vi "Create_AO_Z_WF.vi"(8 "error in":errorcluster) -> (0 "error out":errorcluster)   [LabVIEW 2025]
uses:
  <vilib>/Waveform/WDTOps.llb/WDT Append Waveforms DBL.vi
panel:
  out "Illumination analog waveforms":waveform(dbl)(graph) caption="Output Waveform"
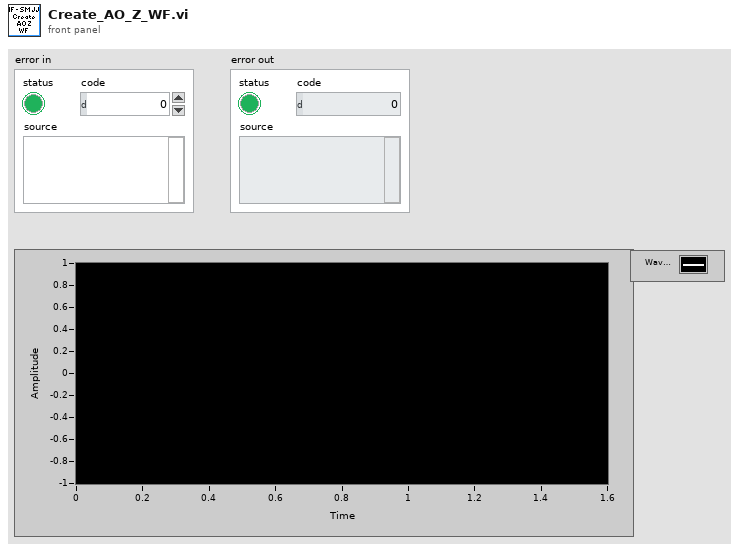
[diagram p1: front panel]
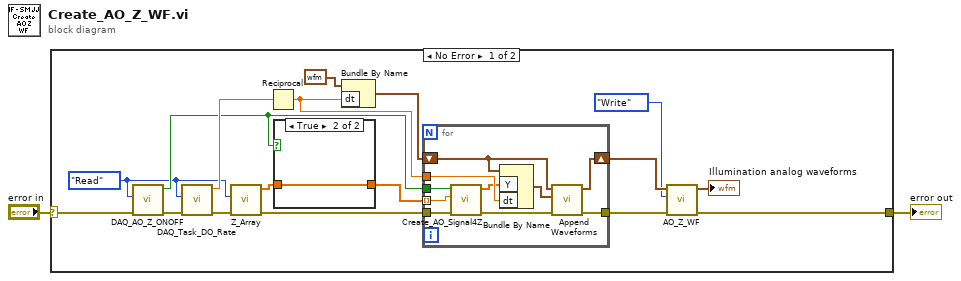
[diagram p0: block diagram]
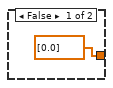
[diagram p2: hidden frame]
diagram:
  n1 = case shown="No Error" "error in" {
    selector: "error in" -> [w19 w32]
    tunnel: [w18 w32] -> w1
    frame No Error {
      w5 = enum16{"Init", "Write", "Read"}."Read" ("Action")
      n2 = call "DAQ_AO_Z_ONOFF.vi"("error in"=w19, "Action"=w5) -> ("error out"=w17:errorcluster, "ON / OFF"=w6:bool)  [unwired: 8 in]
      n3 = call "DAQ_Task_DO_Rate.vi"("error in"=w17, "Action"=w5) -> ("error out"=w9:errorcluster, "DO_Rate"=w16:dbl)  [unwired: 8 in]
      n4 = call "Z_Array.vi"("error in"=w9, "Action"=w5) -> ("error out"=w3:errorcluster, "Z_Array"=w7:dbl[])  [unwired: 8 in]
      n5 = Reciprocal(x=w16) -> (1/x=w13:dbl)
      n6 = case shown="True" w6 {
        tunnel: w7 -> [_ w21]
        tunnel: [dbl[] [0.0] w21] -> w4
        frame False {
        }
        frame True {
        }
      }
      n7 = Bundle By Name(cluster=waveform(dbl) {"t0"=timestamp(0 s since 1904-01-01), "dt"=0.001, "Y"=[]} ("waveform out"), "dt"=w13) -> (w12:waveform(dbl))
      n8 = for {
        tunnel: [w24] -> w10
        tunnel: w6 -> [w31]
        tunnel: w13 -> [w30]
        tunnel: w4 -> [w28] mode=indexing
        tunnel: w3 -> [w27]
        shift-right: [w25] -> w11
        shift-left: w12 -> [w22]
        n9 = call "Create_AO_Signal4Z.vi"("error in"=w27, "AO Amplitude"=w28, "ON / OFF"=w31) -> ("error out"=w26:errorcluster, "WF"=w29:dbl[])  [unwired: 7 in]
        n10 = Bundle By Name(cluster=w22, "Y"=w29, "dt"=w30) -> (w23:waveform(dbl))
        n11 = call-poly <vilib>:"Append Waveforms.vi"("error in (no error)"=w26, "waveform B"=w23, "waveform A"=w22) -> ("error out"=w24:errorcluster, "waveform out"=w25:waveform(dbl))  [unwired: 7 in]
      }
      n12 = call "AO_Z_WF.vi"("error in"=w10, "Action"=enum16{"Init", "Write", "Read"}."Write", "AO Z WF"=w11) -> ("error out"=w18:errorcluster, "AO Z WF"=→"Illumination analog waveforms":waveform(dbl))  [unwired: 7 in]
    }
    frame Error {
    }
  }
  "error out" <- w1
